vi "RingToAmp.vi"(11 "Electrode":T1 {"Magnitude" format="%4.2f"}) -> (3 "Amplitude":sgl)   [LabVIEW 2012, in "StimulCtrls.lvlib"]
uses:
  StimulCtrls.lvlib
  ElectdPanel.ctl
  ElectdTerminal.ctl
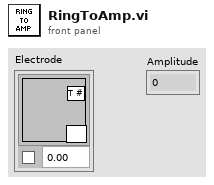
[diagram p1: front panel]
types:
  T1 = typedef "StimulCtrls.lvlib/ElectdPanel.ctl" = cluster{"Group #":string, "T #":T2, "Magnitude":sgl, "Set Voltage":bool}
  T2 = typedef "StimulCtrls.lvlib/ElectdTerminal.ctl" = u8
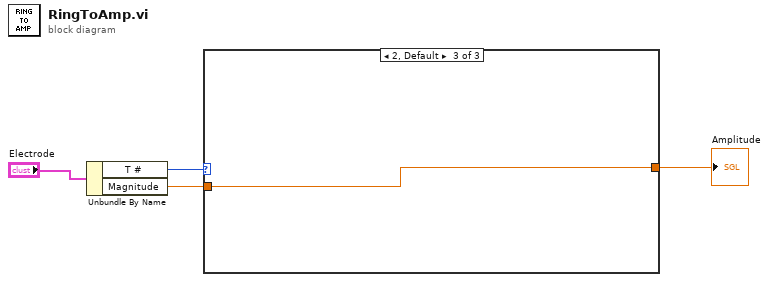
[diagram p0: block diagram]
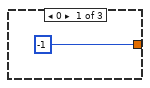
[diagram p2: hidden frame]
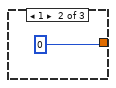
[diagram p3: hidden frame]
diagram:
  n1 = Unbundle By Name("Electrode") -> ("T #"=w3:T2, "Magnitude"=w1:sgl)
  n2 = case shown="2, Default" w3 {
    tunnel: [-1 0 w7] -> w2
    tunnel: w1 -> [_ _ w7]
    frame 0 {
    }
    frame 1 {
    }
    frame 2, Default {
    }
  }
  "Amplitude" <- w2
